vi "isHome.vi"(9 "HomeDetected last state":i32, 10 "Counter last state":i32, 11 "Home area detected":bool) -> (2 "Counter":i32, 3 "HomeDetected=1":i32)   [LabVIEW 2020]
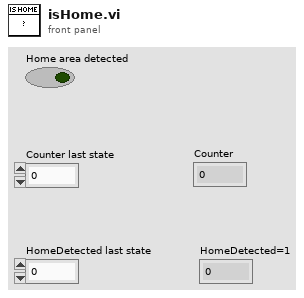
[diagram p1: front panel]
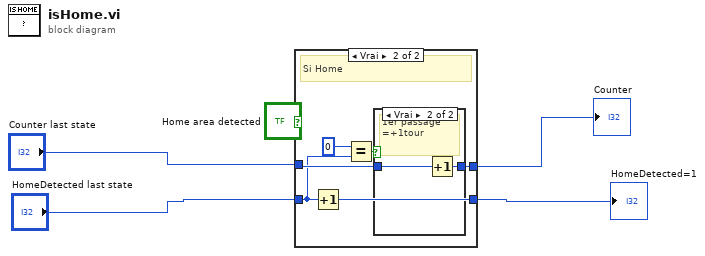
[diagram p0: block diagram]
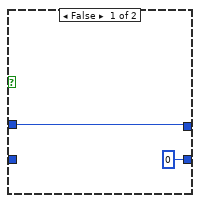
[diagram p2: hidden frame]
diagram:
  n1 = case shown="Vrai" "Home area detected" {
    tunnel: "Counter last state" -> [w7 w13]
    tunnel: [w7 w12] -> w2
    tunnel: "HomeDetected last state" -> [_ w9]
    tunnel: [0 w11] -> w3
    frame False {
    }
    frame True {
      # "Si Home"
      n2 = Increment(x=w9) -> (x+1=w11:i32)
      n3 = Equal?(x=0, y=w9) -> (x = y?=w10:bool)
      n4 = case shown="Vrai" w10 {
        tunnel: w13 -> [w14 w16]
        tunnel: [w14 w15] -> w12
        frame False {
        }
        frame True {
          # "1er passage\n=+1tour"
          n5 = Increment(x=w16) -> (x+1=w15:i32)
        }
      }
    }
  }
  "HomeDetected=1" <- w3
  "Counter" <- w2
